vi "Ctor.vi"(8 "error in (no error)":errorcluster, 11 "ArrayPanel in":refnum<class "ArrayPanel.lvclass">) -> (0 "error out":errorcluster, 3 "ArrayPanel out":refnum<class "ArrayPanel.lvclass">)   [LabVIEW 2014, in "OOPanel.lvlib" / "ArrayPanel.lvclass"]
uses:
  ArrayPanel.lvclass
  Ref Data.ctl
  Panel/Panel.lvclass
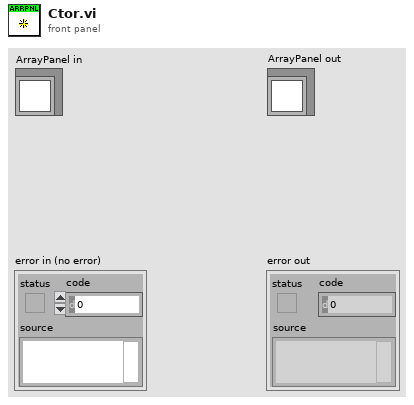
[diagram p1: front panel]
types:
  T1 = typedef "OOPanel.lvlib/ArrayPanel.lvclass/Ref Data.ctl" = cluster{"Orphan":bool}
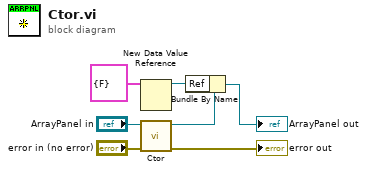
[diagram p0: block diagram]
diagram:
  n1 = New Data Value Reference(data value=T1 {"Orphan"=FALSE} ("Ref Data")) -> (data value reference=w2:refnum<data-value>)  [unwired: 1 in, 1 out]
  n2 = call-parent "Ctor.vi"("error in (no error)"="error in (no error)", "Panel in"="ArrayPanel in") -> ("error out"=→"error out":errorcluster, "Panel out"=w3:refnum<class "ArrayPanel.lvclass">)  [unwired: 8 in]
  n3 = Bundle By Name(cluster=w3, "Ref"=w2) -> (→"ArrayPanel out":refnum<class "ArrayPanel.lvclass">)
